vi "Read from Port.vi"(8 "error in":errorcluster, 10 "TEC Cmd":T1, 11 "TE Cooler in":refnum<class "TE Cooler.lvclass">) -> (0 "error out":errorcluster, 1 "outputStr":string, 2 "scaledOut":sgl, 3 "TE Cooler out":refnum<class "TE Cooler.lvclass">)   [LabVIEW 2018, in "TE Cooler.lvlib" / "TE Cooler.lvclass"]
doc: "Send a command and read the resulting data out. From the manual:\n\nTo write a command to the controller, the controlling computer must send the following ASCII characters:\n(stx)00CCDDDDDDDDSS(etx)\n\nHere, 00 is the only acceptable address for the TC-36-25; CC are the command characters; DDDDDDDD is the ASCII representation of the hexadecimal return or send value. Negative numbers are represented by the hex 2fs complement of the number (32-bit word size):\n 1base10 = 0000000116\n-1base10=ffffffff16"
uses:
  TE Cooler.lvclass
  C:/Users/Labview/Documents/exscalabar_server/Devices/Configurable Device/Configurable Device.lvclass
  Controls/Command.ctl
  Configurable Device/Configurable Device.lvclass/Configurable Device.ctl
  Configurable Device/Accessors/Read Addr.vi
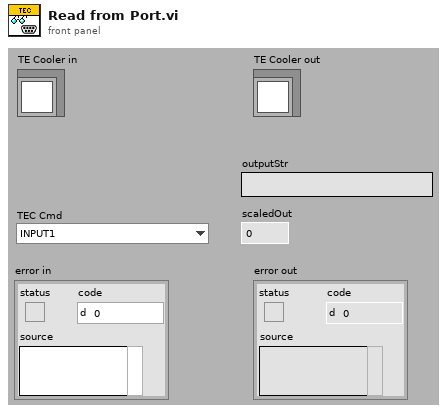
[diagram p1: front panel]
types:
  T1 = typedef "TE Cooler.lvlib/TE Cooler.lvclass/Command.ctl" = enum16{"INPUT1", "DESIRED CONTROL VALUE", "POWER OUTPUT", "ALARM STATUS", "INPUT 2", "OUTPUT CURRENT COUNTS", "ALARM TYPE", "SET TYPE DEFINE", "SENSOR TYPE", "CONTROL TYPE", "CONTROL OUTPUT POLARITY", "POWER ON/OFF", "OUTPUT SHUTDOWN IF ALARM", "FIXED DESIRED CONTROL SETTING", "PROPORTIONAL BANDWIDTH", "INTEGRAL GAIN", "DERIVATIVE GAIN", "LOW EXTERNAL SET RANGE", "HIGH EXTERNAL SET RANGE", "ALARM DEADBAND", "HIGH ALARM SETTING", "LOW ALARM SETTING", "CONTROL DEADBAND SETTING", "INPUT1 OFFSET", "INPUT2 OFFSET", "HEAT MULTIPLIER", "COOL MULTIPLIER", "OVER CURRENT COUNT COMPARE VALUE", "ALARM LATCH ENABLE", "NOT USED", "ALARM LATCH RESET", "CHOOSE SENSOR FOR ALARM FUNCTION", "CHOOSE TEMPERATURE WORKING UNITS", "EEPROM WRITE ENABLE", "OVER CURRENT CONTINUOUS", "OVER CURRENT RESTART ATTEMPTS", "JP3 DISPLAY ENABLE"}
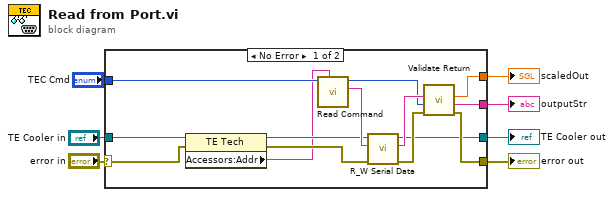
[diagram p0: block diagram]
diagram:
  n1 = case shown="No Error" "error in" {
    selector: "error in" -> [w11 w23]
    tunnel: [w17 w23] -> w6
    tunnel: [w16 w22] -> w4
    tunnel: "TE Cooler in" -> [w12 w22]
    tunnel: [w15 _] -> w3
    tunnel: [w14 _] -> w2
    tunnel: "TEC Cmd" -> [w13 _]
    frame No Error {
      n2 = property class="TE Tech"(reference=w12, error in=w11) -> (reference out=w10:refnum<class "TE Cooler.lvclass">, error out=w9:errorcluster, "Accessors:Addr"=w8:string)
      n3 = call "Read Command.vi"("Addr"=w8, "TEC Cmd"=w13) -> ("String"=w21:string, "Numeric"=w18:i32)  [unwired: 8 in]
      n4 = call "R_W Serial Data.vi"("error in (no error)"=w9, "String In"=w21, "TE Cooler in"=w10) -> ("error out"=w19:errorcluster, "String Out"=w20:string, "TE Cooler out"=w16:refnum<class "TE Cooler.lvclass">)  [unwired: 6 in]
      n5 = call "Validate Return.vi"("error in"=w19, "Divisor"=w18, "Rtn Str"=w20) -> ("error out"=w17:errorcluster, "outputStr"=w14:string, "Output Value"=w15:sgl)  [unwired: 6 in]
    }
    frame Error {
    }
  }
  "error out" <- w6
  "TE Cooler out" <- w4
  "scaledOut" <- w3
  "outputStr" <- w2
